vi "Set Internal Timing Source.vi"(10 "Internal Timing Source":string, 11 "TimerDRV in":refnum<class "TimerDRV.lvclass">) -> (3 "TimerDRV out":refnum<class "TimerDRV.lvclass">)   [LabVIEW 2019, in "TimingDRV Engine.lvlib" / "TimerDRV.lvclass"]
uses:
  TimerDRV.lvclass
  TimerDRV.lvclass/TimerDRV.ctl
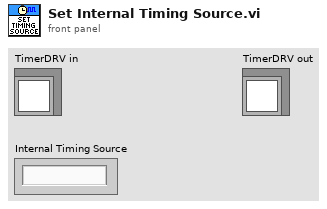
[diagram p1: front panel]
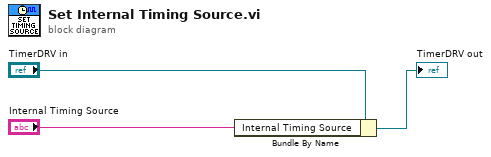
[diagram p0: block diagram]
diagram:
  n1 = Bundle By Name(cluster="TimerDRV in", "Internal Timing Source"="Internal Timing Source") -> (→"TimerDRV out":refnum<class "TimerDRV.lvclass">)
